vi "HXQ-局部-创建特征检测矩形区域A.vi"(4 "方向角":dbl, 5 "产品参考半径":dbl=100.0 format="%#_13g", 6 "底边到ROI左边偏移":dbl=0.05 format="%#_13g", 7 "高径比参数值":dbl=0.6, 8 "矩形ROI半宽比例":dbl=0.1 format="%#_13g", 9 "矩形ROI半长比例":dbl=0.17 format="%#_13g", 10 "Y Resolution":i32, 11 "X Resolution":i32) -> (1 "Height":dbl, 2 "Width":dbl, 3 "矩形输出":cluster{dbl, dbl, dbl, dbl, dbl})   [LabVIEW 2018]
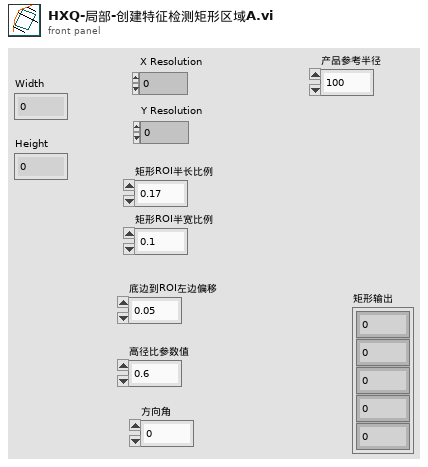
[diagram p1: front panel]
types:
  T1 = typedef "IMAQ Rectangle" = cluster{"Left":i32, "Top":i32, "Right":i32, "Bottom":i32, "Rotation":dbl}
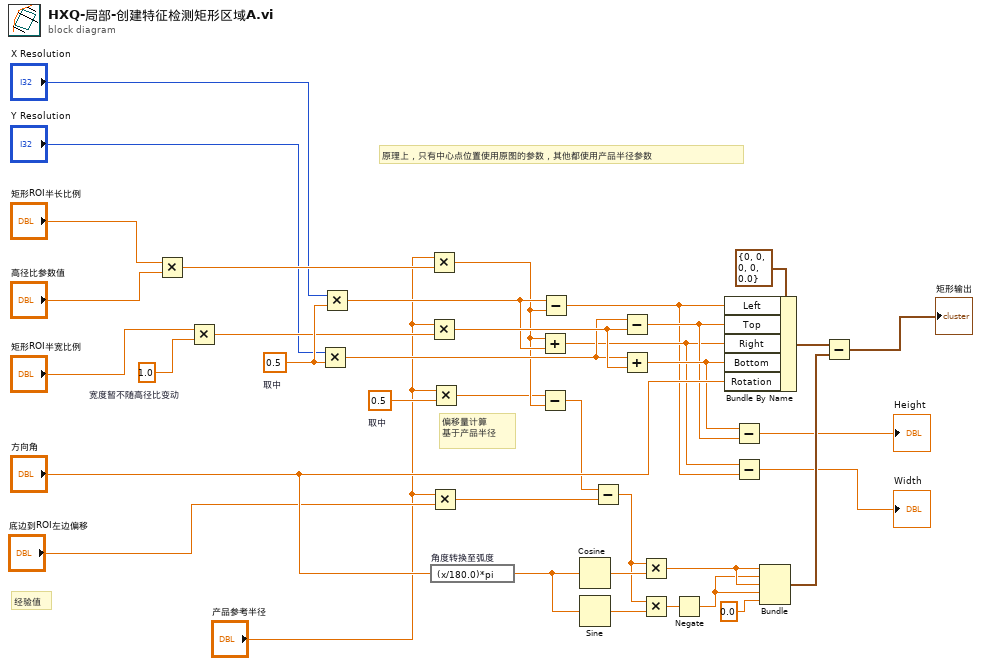
[diagram p0: block diagram]
diagram:
  w8 = 0.5  # 取中
  w18 = 1.0  # 宽度暂不随高径比变动
  w37 = 0.5  # 取中
  # "原理上，只有中心点位置使用原图的参数，其他都使用产品半径参数"
  # "偏移量计算\n基于产品半径"
  # "经验值"
  n1 = Multiply(x="矩形ROI半长比例", y="高径比参数值") -> (x*y=w29:dbl)
  n2 = Multiply(x="矩形ROI半宽比例", y=w18) -> (x*y=w32:dbl)
  n3 = Multiply(x="Y Resolution", y=w37) -> (x*y=w34:dbl)
  n4 = Multiply(x="X Resolution", y=w37) -> (x*y=w35:dbl)
  n5 = Multiply(x="产品参考半径", y=w29) -> (x*y=w11:dbl)
  n6 = Multiply(x="产品参考半径", y=w32) -> (x*y=w36:dbl)
  n7 = Multiply(x="产品参考半径", y="底边到ROI左边偏移") -> (x*y=w16:dbl)
  n8 = Multiply(x="产品参考半径", y=w8) -> (x*y=w9:dbl)
  n9 = expression code="(x/180.0)*pi" "角度转换至弧度"("方向角") -> (w26:dbl)
  n10 = Add(x=w11, y=w35) -> (x+y=w3:dbl)
  n11 = Subtract(x=w9, y=w11) -> (x-y=w10:dbl)
  n12 = Subtract(x=w35, y=w11) -> (x-y=w2:dbl)
  n13 = Cosine(x=w26) -> (cos(x)=w28:dbl)
  n14 = Sine(x=w26) -> (sin(x)=w27:dbl)
  n15 = Subtract(x=w10, y=w16) -> (x-y=w15:dbl)
  n16 = Subtract(x=w34, y=w36) -> (x-y=w5:dbl)
  n17 = Add(x=w34, y=w36) -> (x+y=w6:dbl)
  n18 = Multiply(x=w15, y=w28) -> (x*y=w24:dbl)
  n19 = Multiply(x=w15, y=w27) -> (x*y=w20:dbl)
  n20 = Negate(x=w20) -> (-x=w19:dbl)
  n21 = Bundle By Name(cluster=T1 {"Left"=0, "Top"=0, "Right"=0, "Bottom"=0, "Rotation"=0.0} ("Rectangle"), "Left"=w2, "Top"=w5, "Right"=w3, "Bottom"=w6, "Rotation"="方向角") -> (w22:T1)
  n22 = Subtract(x=w6, y=w5) -> (x-y=→"Height":dbl)
  n23 = Subtract(x=w3, y=w2) -> (x-y=→"Width":dbl)
  n24 = Bundle(w24, w19, w24, w19, "y"=0.0) -> (w21:cluster{dbl, dbl, dbl, dbl, "y":dbl})  [unwired: 1 in]
  n25 = Subtract(x=w22, y=w21) -> (x-y=→"矩形输出":cluster{dbl, dbl, dbl, dbl, dbl})
